vi "compiledEvent.vi"(8 "error in (no error)":errorcluster, 9 "current time":timestamp, 10 "Path":path, 11 "Compiler in":refnum<class "Compiler.lvclass">) -> (0 "error out":errorcluster, 3 "Compiler out":refnum<class "Compiler.lvclass">)   [LabVIEW 2009, in "Compiler.lvlib" / "Compiler.lvclass"]
uses:
  Compiler.lvclass
  Compiler.lvclass/Compiler.ctl
  Hal/HWController/HWControllerEvents/HWControllerEvents.lvclass
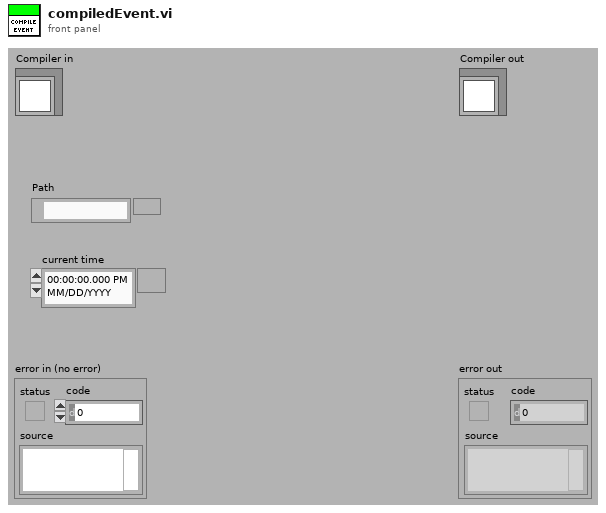
[diagram p1: front panel]
types:
  T1 = enum16{"start", "stop", "statusInquiry", "configure", "resetError", "resourcesInquiry", "reserveResources", "initialise", "resetAllChannels", "staticUpdate", "close", "HWStatus", "error", "resourcesAvailable", "resourcesReserved", "compilerError", "compiledScript", "compilingScript", "runScript", "configureCompiledScript"}
  T2 = cluster{"incomingEventTypes":cluster{"start":cluster{"Boolean":bool}, "stop":cluster{"Boolean":bool}, "statusInquiry":cluster{"Boolean":bool}, "configure":cluster{"DPScriptPath":path, "TimeStamp":string, "HWLoop?":bool}, "resetError":cluster{"Boolean":bool}, "resourcesInquiry":cluster{"Boolean":bool}, "reserveResources":cluster{"HWList":string[]}, "initialise":cluster{"HWList":string[]}, "close":cluster{"Boolean":bool}, "resetAllChannels":cluster{"Boolean":bool}, "staticChannelUpdate":cluster{"channel_address":string, "calibratedValue":dbl}, "runScript":cluster{"DPScriptPath":path, "TimeStamp":string, "HWLoop?":bool}, "compilingScript":cluster{"Path":path}, "compiledScript":cluster{"Path":path, "timeCompileAt":string}, "compilerError":cluster{"Path":path}, "configureCompiledScript":cluster{"DPScriptPath":path, "TimeStamp":string, "HWLoop?":bool, "CompiledScript":cluster{"ScriptListCompiler.lvclass":refnum<class "ScriptListCompiler.lvclass">, "aoChannels":refnum<class "AnalogOutput.lvclass">[], "doChannels":refnum<class "DigitalOutput.lvclass">[], "rfChannels":refnum<class "DDSOutput.lvclass">[]}}, "restartCompiler":cluster{"restart":bool}, "staticRfChannelUpdate":cluster{"channel_address":string, "Output":cluster{"Frequency(MHz)":dbl, "Amplitude":dbl, "Phase":dbl, "OutputForm":enum16{"Sine", "Square", "Triangle", "Arbitrary"}}}, "cameraUpdate":cluster{"Camera":string, "Type":string, "settings":path}}, "outgoingEventTypes":cluster{"HWStatus":cluster{"status":enum16{"Ready", "Compiling", "Configured", "Running", "Stopping", "Unresolved Error"}}, "error":cluster{"error out":errorcluster}, "resourcesAvailable":cluster{"availableHWList":string[], "reservedHWList":string[]}, "resourcesReserved":cluster{"reservedHWList":string[]}}}
  T3 = cluster{"eventId":enum16{"start", "stop", "statusInquiry", "configure", "resetError", "resourcesInquiry", "reserveResources", "initialise", "resetAllChannels", "staticUpdate", "close", "HWStatus", "error", "resourcesAvailable", "resourcesReserved", "compilerError", "compiledScript", "compilingScript", "runScript", "configureCompiledScript"}, "compiledScript":cluster{"Path":path, "timeCompileAt":string}}
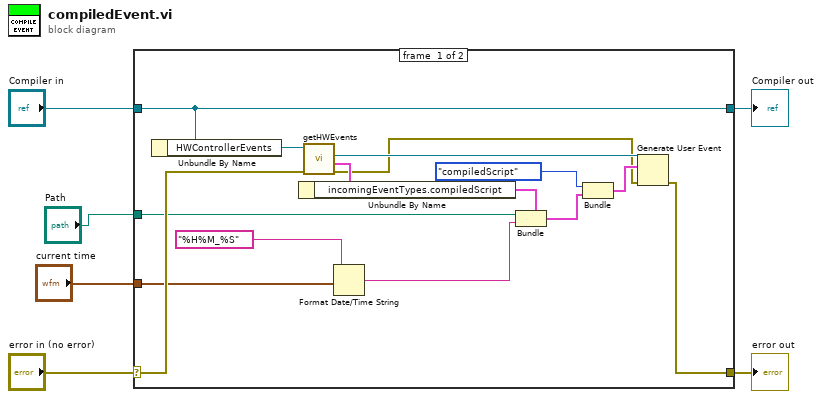
[diagram p0: block diagram]
diagram:
  n1 = case shown="No Error" "error in (no error)" {
    selector: "error in (no error)" -> [w19 w23]
    tunnel: [w10 w23] -> w5
    tunnel: [w21 w22] -> w3
    tunnel: "Compiler in" -> [w21 w22]
    tunnel: "Path" -> [w16 _]
    tunnel: "current time" -> [w9 _]
    frame #0 {
      n2 = Unbundle By Name(w21) -> ("HWControllerEvents"=w20:refnum<class "HWControllerEvents.lvclass">)
      n3 = call-dynamic "getHWEvents.vi"("error in (no error)"=w19, "HWControllerEvents in"=w20) -> ("error out"=w11:errorcluster, "eventDataTypes"=w18:T2, "HWCEvent"=w13:refnum<user-event>)  [unwired: 6 in, 1 out]
      n4 = Unbundle By Name(w18) -> ("incomingEventTypes.compiledScript"=w17:cluster{"Path":path, "timeCompileAt":string})
      n5 = Format Date/Time String(time format string (%c)="%H%M_%S", seconds (now)=w9) -> (date/time string=w7:string)  [unwired: 1 in]
      n6 = Bundle(cluster=w17, "Path"=w16, "timeCompileAt"=w7) -> (w15:cluster{"Path":path, "timeCompileAt":string})
      n7 = Bundle("eventId"=T1."compiledScript", "compiledScript"=w15) -> (w12:T3)  [unwired: 1 in]
      n8 = Generate User Event(user event=w13, event data cluster=w12, error in=w11) -> (error out=w10:errorcluster)  [unwired: 1 out]
    }
    frame #1 {
    }
  }
  "error out" <- w5
  "Compiler out" <- w3
